vi "Adjust_Volt.vi"() -> ()   [LabVIEW 2016, in "Hall Effect Library.lvlib"]
uses:
  Hall Effect Library.lvlib
  Global Variables/Instrument Locations.vi
panel:
  in  "?":bool
  # "Please adjust the potentiometer for a reading of 0V \n on the voltmeter.\n \nIf you finish this process, please press OK button."
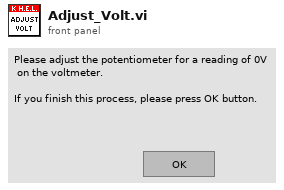
[diagram p1: front panel]
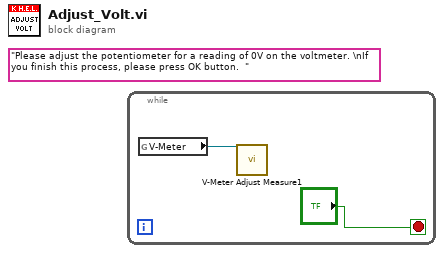
[diagram p0: block diagram]
diagram:
  (unwired) "Please adjust the potentiometer for a reading of 0V on the voltmeter. \nIf you finish this process, please press OK button.  "
  n1 = while {
    stop <- "?" stop-if-true
    n2 = global read "Instrument Locations.vi" "V-Meter"() -> (w1:refnum<visa-resource-name>)
    n3 = call "V-Meter Adjust Measure1.vi"("VISA resource name in"=w1) -> ()  [unwired: 9 in, 2 out]
  }
